vi "Get_Redirect_URI.vi"(8 "error in (no error)":errorcluster, 11 "Asana in":refnum<class "Asana.lvclass">) -> (0 "error out":errorcluster, 3 "Asana out":refnum<class "Asana.lvclass">)   [LabVIEW 2016, in "Asana.lvclass"]
uses:
  Asana.lvclass
  Asana.lvclass/Asana.ctl
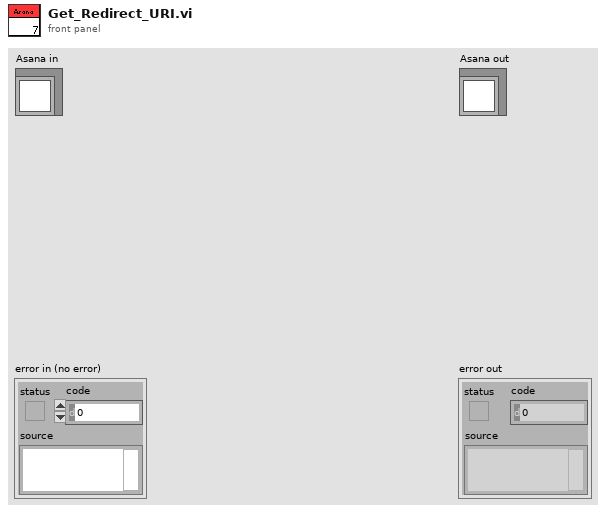
[diagram p1: front panel]
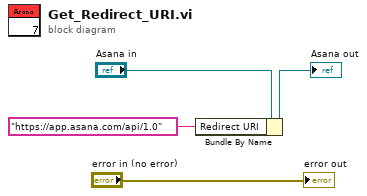
[diagram p0: block diagram]
diagram:
  n1 = Bundle By Name(cluster="Asana in", "Redirect URI"="https://app.asana.com/api/1.0") -> (→"Asana out":refnum<class "Asana.lvclass">)
  "error out" <- "error in (no error)"
